vi "FM Voice Receiver - Save.vi"() -> ()   [LabVIEW 2013]
uses:
  <vilib>/sound2/lvsound2.llb/Sound File Write Open.vi
  <instrlib>/niUSRP/niUSRP Fetch Rx Data (CDB WDT).vi
  <vilib>/Analysis/2dsp.llb/Rational Resample (single channel, DBL).vi
  <vilib>/sound2/lvsound2.llb/Sound File Write (DBL Single).vi
  <vilib>/express/express analysis/Spectral/Block/exnSpectralBlock spectral measurements RMS poly.vi
  <vilib>/express/express analysis/Spectral/Block/exnSpectralBlock spectral measurements RMS WFM.vi
  <vilib>/express/express analysis/Spectral/XNode/ExpressSpectralMeasurementsBlockNode.xnode
  <vilib>/Analysis/NI_AALPro.lvlib
panel:
  in  "Save Path":path=path "E:/07/0416/output.wav"
  out "File Error Out":errorcluster
  in  "Sound Format":T1={"sample rate (S/s)"=44100.0, "number of channels"=1.0, "bits per sample"=16.0}
  out "Spectrum (FFT)":cluster{"f0":dbl, "df":dbl, "magnitude":dbl[]}(graph)
  out "Waveform":waveform(dbl)(graph)
  out "Constellation":cluster{dbl[], dbl[]}(graph)
  out "USRP Error Out":errorcluster
  out "Coerced Gain":dbl format="%#_6f"
  out "Coerced Carrier Freq.":dbl=2400010000.007024 format="%#_6p"
  out "Coerced IQ Rate":dbl=200000.0 format="%#_6p"
  in  "Stop":bool
  in  "Active Antenna":string="RX2"
  in  "Gain":dbl format="%#_6f"
  in  "Carrier Frequency":dbl=1200000000.0 format="%#_6p"
  in  "IQ Rate":dbl=200000.0 format="%#_6p"
  in  "Device Address":refnum<k15>="192.168.10.2"
  in  "Number of Samples":i32=44100
  # "FM Receiver"
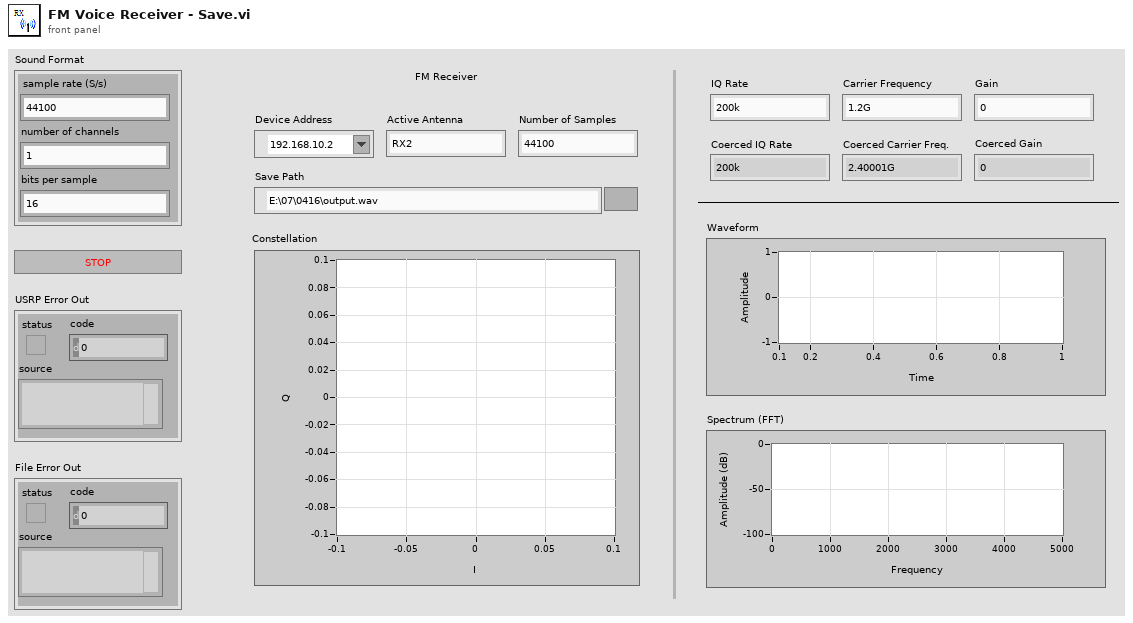
[diagram p1: front panel]
types:
  T1 = cluster{"sample rate (S/s)":dbl, "number of channels":dbl, "bits per sample":dbl}
  T2 = typedef "Sound File Refnum.ctl" = refnum<file>
  T3 = cluster{"averaging mode":u16, "weighting mode":u16, "number of averages":u32}
  T4 = cluster{"dB On (F)":bool, "unwrap phase (F)":bool, "convert to degree (F)":bool}
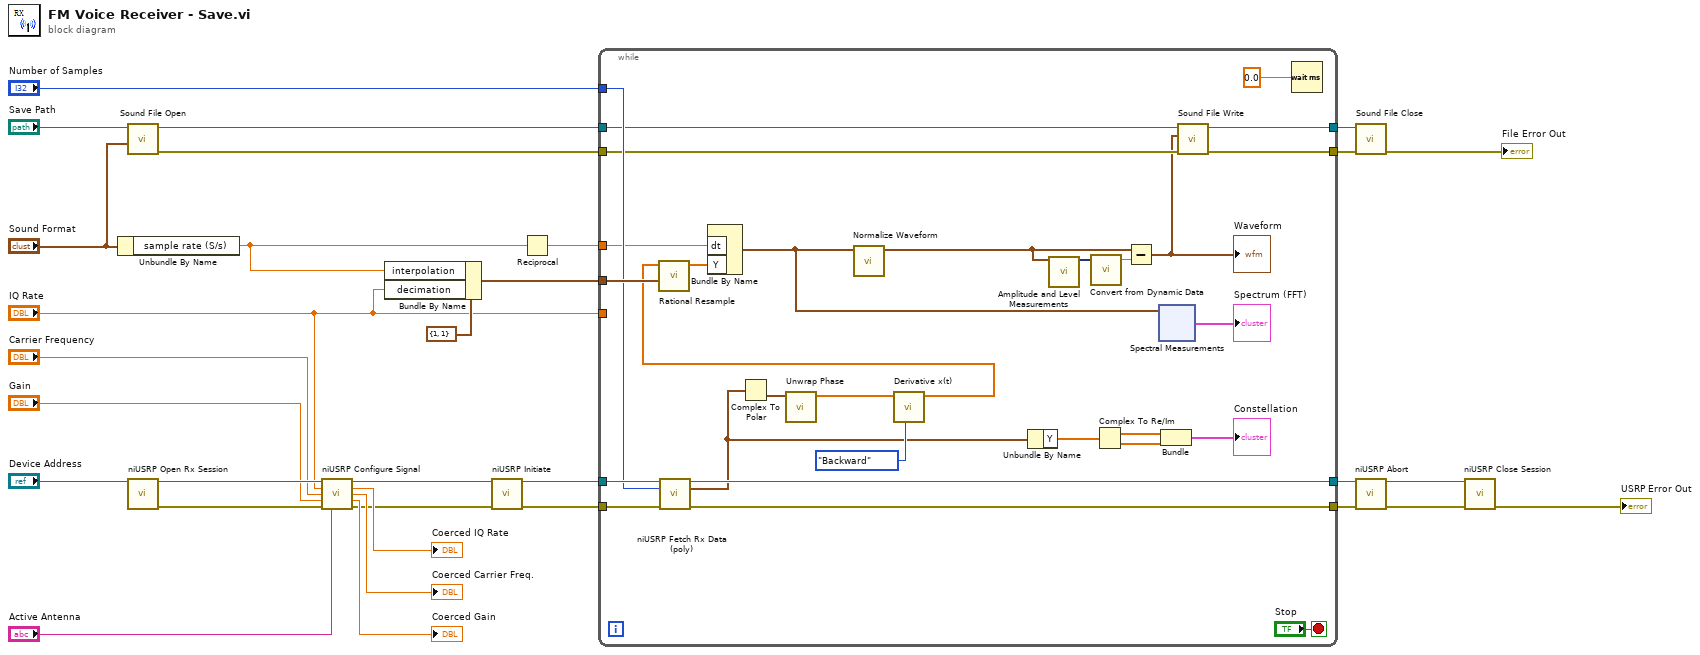
[diagram p0: block diagram]
diagram:
  n1 = Unbundle By Name("Sound Format") -> ("sample rate (S/s)"=w13:dbl)
  n2 = call-poly <vilib>:"Sound File Open.vi"("sound format"="Sound Format", "path"="Save Path") -> ("error out"=w6:errorcluster, "sound file refnum"=w7:T2)  [unwired: 8 in]
  n3 = call <instrlib>:"niUSRP Open Rx Session.vi"("device names"="Device Address") -> ("session handle out"=w31:refnum<k15>, "error out"=w30:errorcluster)  [unwired: 13 in]
  n4 = call <instrlib>:"niUSRP Configure Signal.vi"("session handle"=w31, "IQ rate"="IQ Rate", "carrier frequency"="Carrier Frequency", "gain"="Gain", "error in (no error)"=w30, "active antenna"="Active Antenna") -> ("session handle out"=w17:refnum<k15>, "coerced IQ rate"=→"Coerced IQ Rate":dbl, "coerced carrier frequency"=→"Coerced Carrier Freq.":dbl, "coerced gain"=→"Coerced Gain":dbl, "error out"=w15:errorcluster)  [unwired: 5 in]
  n5 = Bundle By Name(cluster=cluster{"decimation":i32, "interpolation":i32} {"decimation"=1, "interpolation"=1}, "interpolation"=w13, "decimation"="IQ Rate") -> (w25:cluster{"decimation":i32, "interpolation":i32})
  n6 = call <instrlib>:"niUSRP Initiate.vi"("session handle"=w17, "error in (no error)"=w15) -> ("session handle out"=w16:refnum<k15>, "error out"=w14:errorcluster)  [unwired: 12 in]
  n7 = Reciprocal(x=w13) -> (1/x=w8:dbl)
  n8 = while {
    tunnel: w16 -> [w60]
    tunnel: [w58] -> w12
    tunnel: [w57] -> w11
    tunnel: w14 -> [w56]
    tunnel: "Number of Samples" -> [w52]
    tunnel: w25 -> [w55]
    tunnel: "IQ Rate" -> [_]
    tunnel: w8 -> [w46]
    tunnel: w7 -> [w36]
    tunnel: w6 -> [w35]
    tunnel: [w34] -> w4
    tunnel: [w33] -> w3
    stop <- "Stop" stop-if-true
    n9 = call-poly <instrlib>:"niUSRP Fetch Rx Data (poly).vi"("session handle"=w60, "number of samples"=w52, "error in (no error)"=w56) -> ("session handle out"=w58:refnum<k15>, "data"=w41:waveform(cdb), "error out"=w57:errorcluster)  [unwired: 9 in, 1 out]
    n10 = Complex To Polar(r * e^(i*theta)=w41) -> (theta=w45:waveform(dbl))  [unwired: 1 out]
    n11 = call <vilib>:"Unwrap Phase.vi"("Phase"=w45) -> ("Unwrapped Phase"=w44:dbl[])  [unwired: 9 in, 1 out]
    n12 = call <vilib>:"Derivative x(t).vi"("method"=enum16{"Backward"}."Backward", "X"=w44) -> ("dX/dt"=w42:dbl[])  [unwired: 8 in, 1 out]
    n13 = call-poly <vilib>:"Rational Resample.vi"("resample factor"=w55, "X"=w42) -> ("Y"=w47:dbl[])  [unwired: 7 in, 2 out]
    n14 = Bundle By Name("dt"=w46, "Y"=w47) -> (w37:waveform(dbl))  [unwired: 1 in]
    n15 = call <vilib>:"Normalize Waveform.vi"("waveform in"=w37) -> ("normalized waveform"=w40:waveform(dbl))  [unwired: 7 in, 3 out]
    n16 = Unbundle By Name(w41) -> ("Y"=w49:cdb[])
    n17 = call "Amplitude and Level Measurements"("Signals"=w40) -> ("Mean (DC)"=w39:dynamicdata)  [unwired: 13 in, 1 out]
    n18 = call "Convert from Dynamic Data"("Dynamic Data Type"=w39) -> ("Scalar"=w38:dbl)  [unwired: 3 in]
    n19 = Complex To Re/Im(x + iy=w49) -> (x=w51:dbl[], y=w50:dbl[])
    n20 = Subtract(x=w40, y=w38) -> (x-y=w32:waveform(dbl))
    "Waveform" <- w32
    n21 = xnode ("Spectral Measurements")("Signals"=w37) -> ("FFT - (RMS)"=→"Spectrum (FFT)":cluster{"f0":dbl, "df":dbl, "magnitude":dbl[]})  [unwired: 1 in, 2 out]
    n22 = Bundle(w51, w50) -> (→"Constellation":cluster{dbl[], dbl[]})  [unwired: 1 in]
    n23 = call-poly <vilib>:"Sound File Write.vi"("error in (no error)"=w35, "data"=w32, "sound file refnum"=w36) -> ("error out"=w33:errorcluster, "sound file refnum out"=w34:T2)  [unwired: 7 in]
    n24 = Wait (ms)(milliseconds to wait=0.0) -> ()  [unwired: 1 out]
  }
  n25 = call <vilib>:"Sound File Close.vi"("error in (no error)"=w3, "sound file refnum"=w4) -> ("error out"=→"File Error Out":errorcluster)  [unwired: 9 in]
  n26 = call <instrlib>:"niUSRP Abort.vi"("session handle"=w12, "error in (no error)"=w11) -> ("session handle out"=w9:refnum<k15>, "error out"=w10:errorcluster)  [unwired: 12 in]
  n27 = call <instrlib>:"niUSRP Close Session.vi"("session handle"=w9, "error in (no error)"=w10) -> ("error out"=→"USRP Error Out":errorcluster)  [unwired: 13 in]
